vi "Verify_Modbus_CRC.vi"(0 "VISA resource name":refnum<visa-resource-name>, 1 "Length":u8, 2 "header":u8[](array[numeric]), 3 "error in (no error)":errorcluster) -> (7 "VISA Refnum out":refnum<visa-resource-name>, 8 "datos del mensaje":T1, 10 "error out":errorcluster)   [LabVIEW 2026]
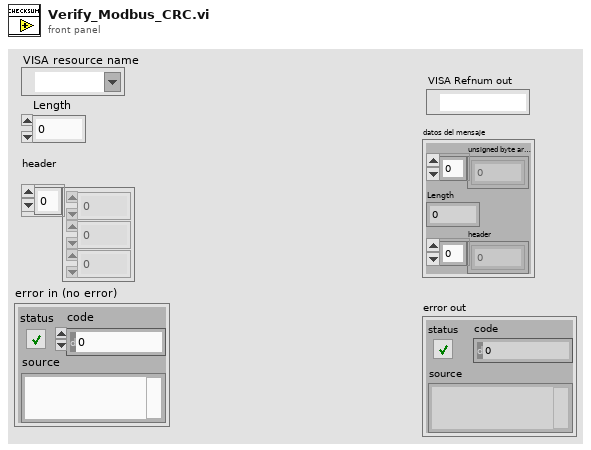
[diagram p1: front panel]
types:
  T1 = cluster{"unsigned byte array":u8[], "Length":u8, "header":u8[]}
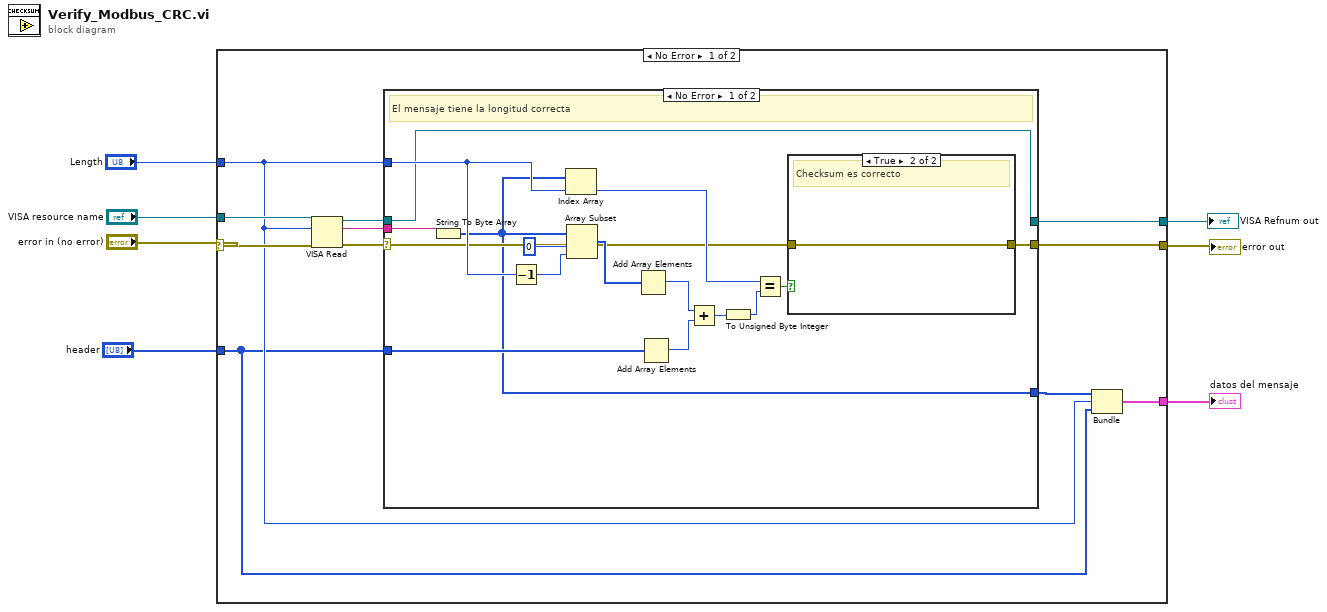
[diagram p0: block diagram]
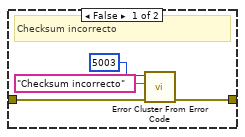
[diagram p2: hidden frame]
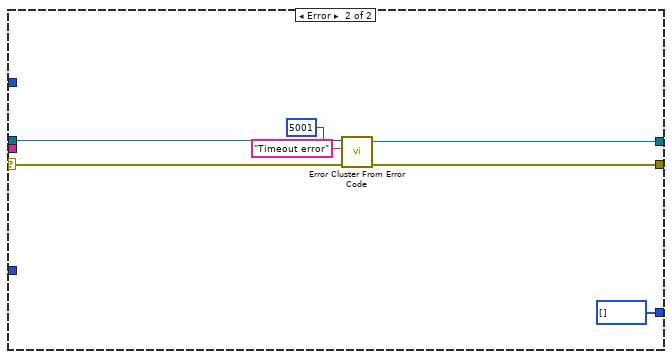
[diagram p3: hidden frame]
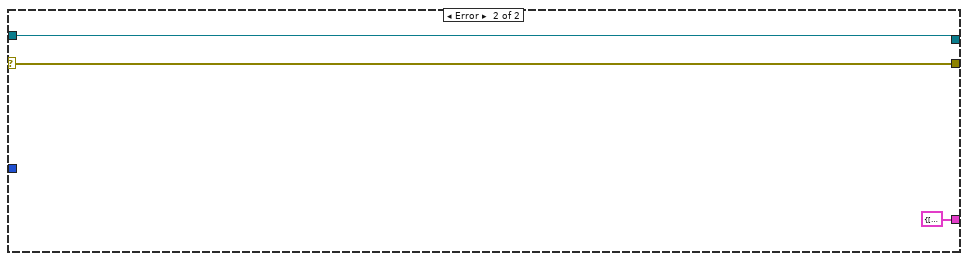
[diagram p4: hidden frame]
diagram:
  n1 = case shown="No Error" "error in (no error)" {
    selector: "error in (no error)" -> [w17 w47]
    tunnel: "VISA resource name" -> [w18 w48]
    tunnel: [w13 w48] -> w5
    tunnel: [w15 w47] -> w4
    tunnel: "Length" -> [w10 _]
    tunnel: "header" -> [w9 _]
    tunnel: [w8 T1 {"unsigned byte array"=[], "Length"=0, "header"=[]}] -> w1
    frame No Error {
      n2 = VISA Read(VISA resource name=w18, byte count=w10, error in (no error)=w17) -> (VISA resource name out=w14:refnum<visa-resource-name>, read buffer=w12:string, error out=w16:errorcluster)  [unwired: 1 out]
      n3 = case shown="No Error" w16 {
        selector: w16 -> [w22 w43]
        tunnel: [w20 w42] -> w15
        tunnel: w14 -> [w21 w41]
        tunnel: [w21 w41] -> w13
        tunnel: w12 -> [w34 _]
        tunnel: w10 -> [w29 _]
        tunnel: w9 -> [w31 _]
        tunnel: [w19 u8[] [] ("unsigned byte array")] -> w11
        frame No Error {
          # "El mensaje tiene la longitud correcta"
          n4 = String To Byte Array(string=w34) -> (unsigned byte array=w19:u8[])
          n5 = Decrement(x=w29) -> (x-1=w30:u8)
          n6 = Index Array(array=w19, index=w29) -> (element=w28:u8)
          n7 = Array Subset(array=w19, index=0, length=w30) -> (w32:u8[])
          n8 = Add Array Elements(numeric array=w32) -> (sum=w27:u8)
          n9 = Add Array Elements(numeric array=w31) -> (sum=w26:u8)
          n10 = Add(x=w27, y=w26) -> (x+y=w25:u8)
          n11 = To Unsigned Byte Integer(number=w25) -> (unsigned 8bit integer=w24:u8)
          n12 = Equal?(x=w28, y=w24) -> (x = y?=w23:bool)
          n13 = case shown="True" w23 {
            tunnel: w22 -> [w35 w39]
            tunnel: [w36 w39] -> w20
            frame False {
              # "Checksum incorrecto"
              n14 = call <vilib>:"Error Cluster From Error Code.vi"("error in (no error)"=w35, "error message (\"\")"="Checksum incorrecto" ("error message (\"\")"), "error code (0)"=5003) -> ("error out"=w36:errorcluster)  [unwired: 6 in]
            }
            frame True {
              # "Checksum es correcto"
            }
          }
        }
        frame Error {
          n15 = call <vilib>:"Error Cluster From Error Code.vi"("error in (no error)"=w43, "error message (\"\")"="Timeout error" ("error message (\"\")"), "error code (0)"=5001) -> ("error out"=w42:errorcluster)  [unwired: 6 in]
        }
      }
      n16 = Bundle("unsigned byte array"=w11, "Length"=w10, "header"=w9) -> (w8:T1)  [unwired: 1 in]
    }
    frame Error {
    }
  }
  "VISA Refnum out" <- w5
  "error out" <- w4
  "datos del mensaje" <- w1
